vi "Create Day of Week.vi"(8 "error in (no error)":errorcluster, 9 "Day":i32, 10 "Month":i32, 11 "Year":i32) -> (0 "error out":errorcluster, 3 "Day of Week":string)   [LabVIEW 2016, in "Environment Chamber.lvlib" / "Climatic Chamber.lvlib"]
uses:
  Climatic Chamber.lvlib
  <vilib>/Utility/miscctls.llb/LVDateTimeRec.ctl
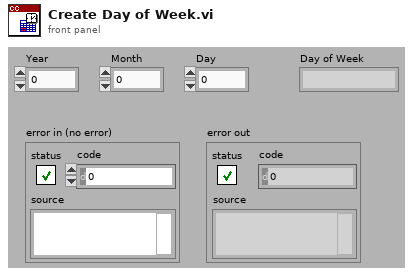
[diagram p1: front panel]
types:
  T1 = typedef "LVDateTimeRec.ctl" = cluster{"fractional second":dbl, "second":i32, "minute":i32, "hour":i32, "day of month":i32, "month":i32, "year":i32, "day of week":i32, "day of year":i32, "DST":i32}
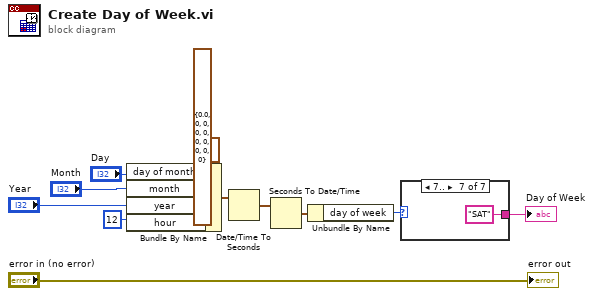
[diagram p0: block diagram]
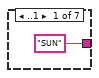
[diagram p2: hidden frame]
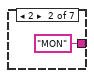
[diagram p3: hidden frame]
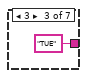
[diagram p4: hidden frame]
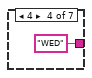
[diagram p5: hidden frame]
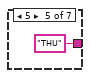
[diagram p6: hidden frame]
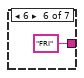
[diagram p7: hidden frame]
diagram:
  n1 = Bundle By Name(cluster=T1 {"fractional second"=0.0, "second"=0, "minute"=0, "hour"=0, "day of month"=0, "month"=0, "year"=0, "day of week"=0, "day of year"=0, "DST"=0} ("date time rec"), "day of month"="Day", "month"="Month", "year"="Year", "hour"=12) -> (w7:T1)
  n2 = Date/Time To Seconds(2:w7) -> (0:w8:timestamp)  [unwired: 1 in]
  n3 = Seconds To Date/Time(time stamp (now)=w8) -> (date time rec=w9:T1)  [unwired: 1 in]
  n4 = Unbundle By Name(w9) -> ("day of week"=w10:i32)
  n5 = case shown="7.." w10 {
    tunnel: ["SUN" "MON" "TUE" "WED" "THU" "FRI" "SAT"] -> w11
    frame ..1 {
    }
    frame 2 {
    }
    frame 3 {
    }
    frame 4 {
    }
    frame 5 {
    }
    frame 6 {
    }
    frame 7.. {
    }
  }
  "Day of Week" <- w11
  "error out" <- "error in (no error)"
